vi "try_Random Number in Range.vi"() -> ()   [LabVIEW 2020]
uses:
  <vilib>/numeric/Random Number (Range) DBL.vi
panel:
  out "Waveform Graph":dbl[](graph)
  out "Array":dbl[](array[numeric])
  in  "Number of Array Elements":i32=300
  in  "Lower Bound":dbl=-3.14159
  in  "Upper Bound":dbl=127.0
  # "Scenario\nThe Random Number (Range).vi allows you to generate a random number between a minimum and maximum specified value\n\nInstructions\n1. Set the Upper Bound, Lower Bound, and Number of Array Elements \n2. Run the VI"
  # "Close this VI when you are done with the demo."
  # "You do not need to save changes to this VI."
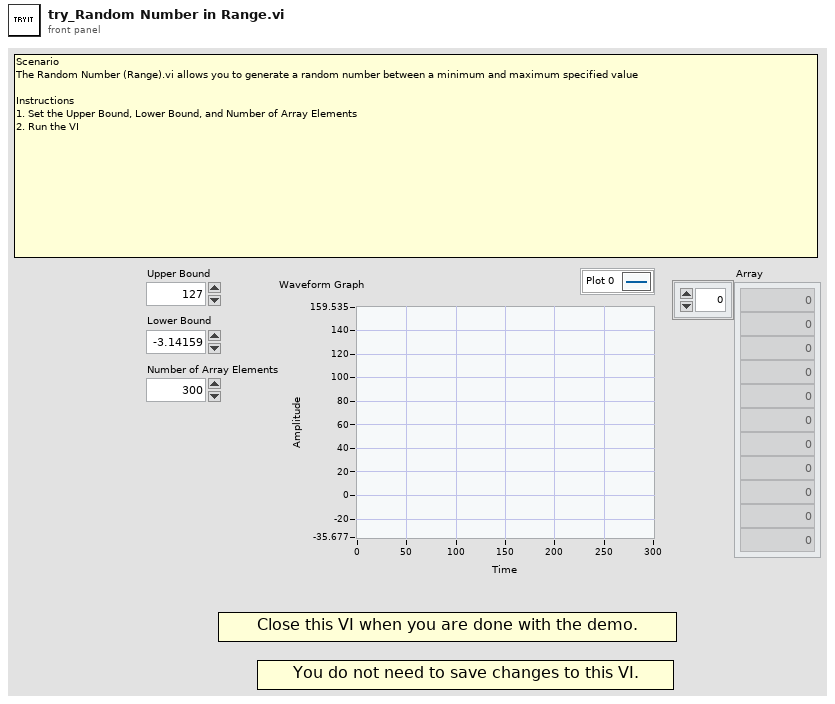
[diagram p1: front panel]
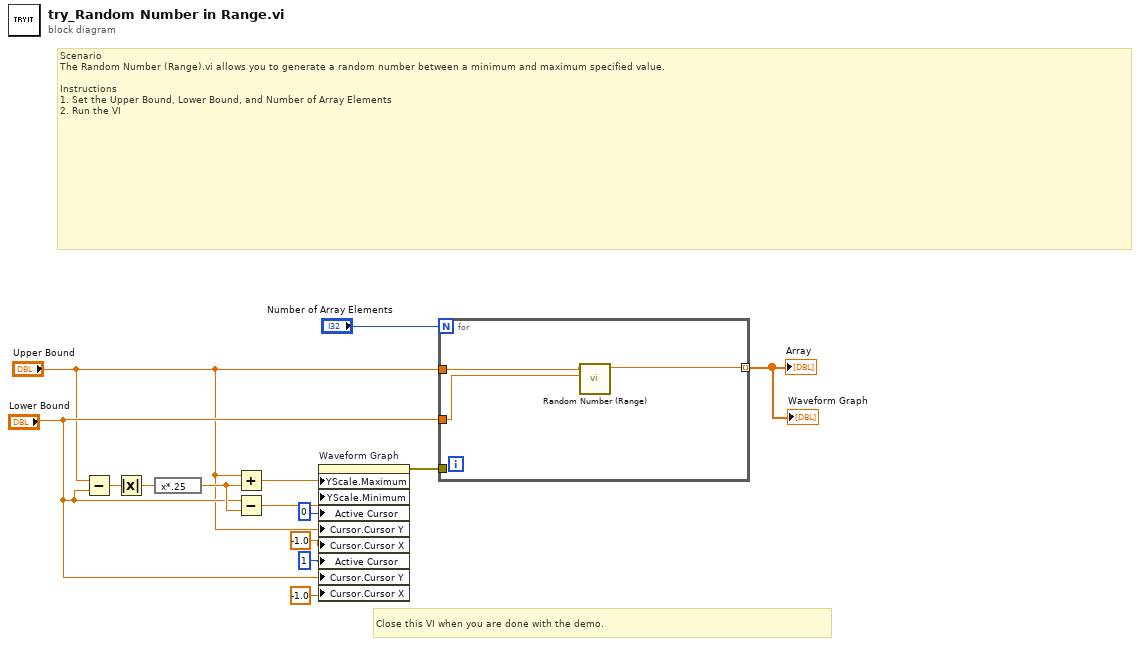
[diagram p0: block diagram]
diagram:
  # "Close this VI when you are done with the demo."
  # "Scenario\nThe Random Number (Range).vi allows you to generate a random number between a minimum and maximum specified value.\n\nInstructions\n1. Set the Upper Bound, Lower Bound, and Number of Array Elements \n2. Run the VI"
  n1 = Subtract(x="Upper Bound", y="Lower Bound") -> (x-y=w7:dbl)
  n2 = Absolute Value(x=w7) -> (abs(x)=w6:dbl)
  n3 = expression code="x*.25"(w6) -> (w3:dbl)
  n4 = Add(x="Upper Bound", y=w3) -> (x+y=w5:dbl)
  n5 = Subtract(x="Lower Bound", y=w3) -> (x-y=w4:dbl)
  n6 = property on="Waveform Graph" class="WFGraph (strict)"("YScale.Maximum"=w5, "YScale.Minimum"=w4, "Active Cursor"=u32 0, "Cursor.Cursor Y"="Upper Bound", "Cursor.Cursor X"=-1.0 ("Cursor.Cursor Position:Cursor X"), "Active Cursor"=u32 1, "Cursor.Cursor Y"="Lower Bound", "Cursor.Cursor X"=-1.0 ("Cursor.Cursor Position:Cursor X")) -> (error out=w8:errorcluster)  [unwired: 2 in, 1 out]
  n7 = for {
    N: "Number of Array Elements" -> [_]
    tunnel: "Upper Bound" -> [w17]
    tunnel: "Lower Bound" -> [w16]
    tunnel: [w15] -> w13 mode=indexing
    tunnel: w8 -> [_]
    n8 = call-poly <vilib>:"Random Number (Range).vi"("lower bound (0)"=w16, "upper bound (100)"=w17) -> ("number"=w15:dbl)  [unwired: 9 in]
  }
  "Array" <- w13
  "Waveform Graph" <- w13
